vi "SetSpeed.vi"(8 "error in (no error)":errorcluster, 10 "Speed":i32, 11 "reference in":refnum<class "CeilingFan.lvclass">) -> (0 "error out":errorcluster, 3 "reference out":refnum<class "CeilingFan.lvclass">)   [LabVIEW 2020, in "CeilingFan.lvclass"]
uses:
  CeilingFan.lvclass
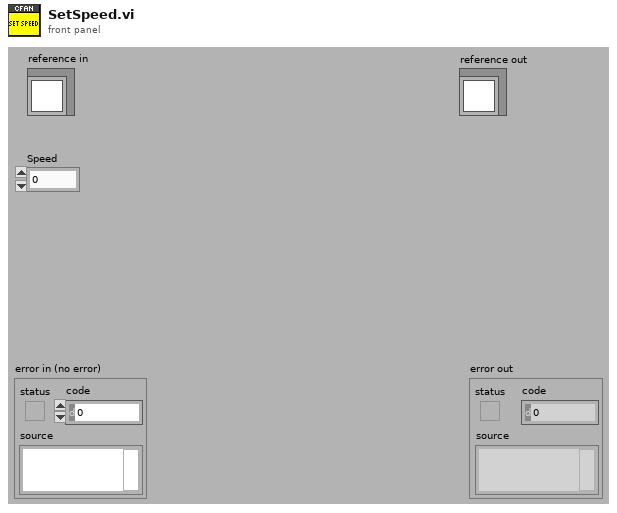
[diagram p1: front panel]
types:
  T1 = typedef "CeilingFan.lvclass/ObjectAttributes.ctl" = cluster{"Speed":i32}
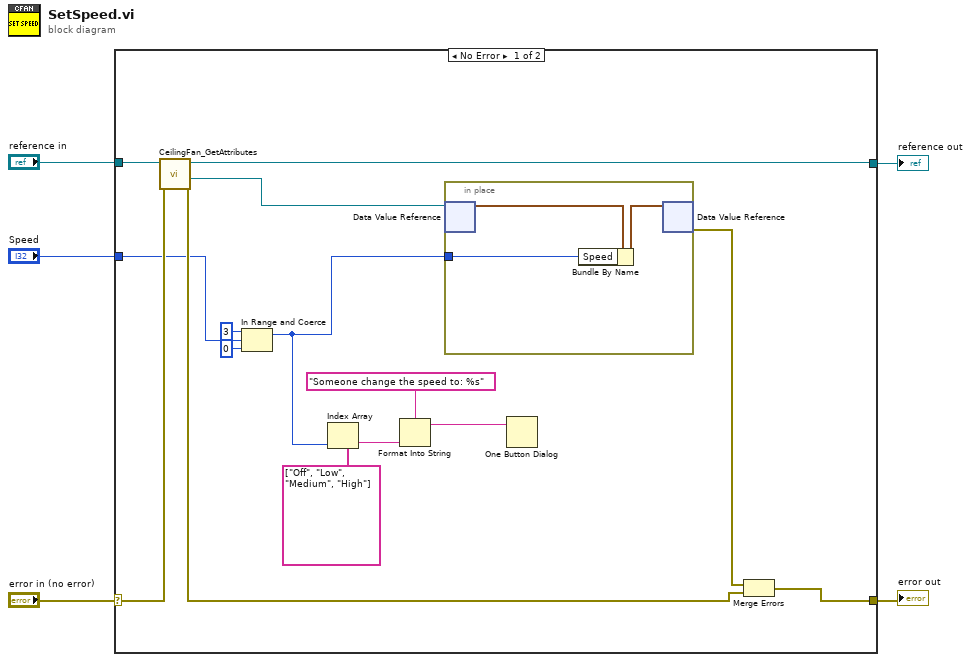
[diagram p0: block diagram]
diagram:
  n1 = case shown="No Error" "error in (no error)" {
    selector: "error in (no error)" -> [w15 w25]
    tunnel: [w19 w25] -> w4
    tunnel: [w17 w24] -> w2
    tunnel: "reference in" -> [w18 w24]
    tunnel: "Speed" -> [w11 _]
    frame No Error {
      n2 = call "CeilingFan_GetAttributes.vi"("error in (no error)"=w15, "reference in"=w18) -> ("error out"=w14:errorcluster, "DataRef"=w16:refnum<data-value>, "reference out"=w17:refnum<class "CeilingFan.lvclass">)  [unwired: 6 in, 1 out]
      n3 = In Range and Coerce(upper limit=3, x=w11, lower limit=0) -> (coerced(x)=w10:i32)  [unwired: 1 out]
      n4 = Index Array(array=string[] ["Off", "Low", "Medium", "High"], index=w10) -> (element=w8:string)
      n5 = Format Into String(format string="Someone change the speed to: %s" ("TextIn"), w8) -> (resulting string=w6:string)  [unwired: 2 in, 1 out]
      n6 = in-place {
        in-place-border: w10 -> [w23]
        n7 = in-place-dvr #1(w16) -> (w22:T1)  [unwired: 1 out]
        n8 = Bundle By Name(cluster=w22, "Speed"=w23) -> (w21:T1)
        n9 = in-place-dvr #1(w21) -> (w20:errorcluster)  [unwired: 1 out]
      }
      n10 = One Button Dialog(message=w6) -> ()  [unwired: 1 in, 1 out]
      n11 = Merge Errors(w20, w14) -> (w19:errorcluster)
    }
    frame Error {
    }
  }
  "error out" <- w4
  "reference out" <- w2
